vi "Check For Errors.vi"(8 "Error In":errorcluster, 11 "Process In":refnum<class "Process.lvclass">) -> (0 "Error Out":errorcluster, 2 "Error Detected":bool, 3 "Process Out":refnum<class "Process.lvclass">)   [LabVIEW 2021, in "Process.lvclass"]
uses:
  Process.lvclass
  Central Message Handler/Public/Controls/Message.ctl
  Central Message Handler/Central Message Handler.lvclass
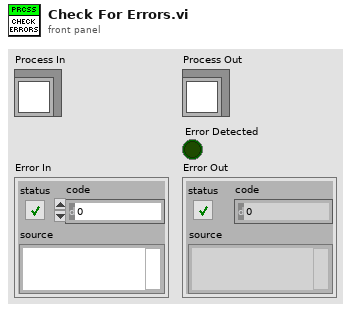
[diagram p1: front panel]
types:
  T1 = typedef "Central Message Handler.lvclass/Message.ctl" = cluster{"Command":string, "Data":variant, "Receiver":string}
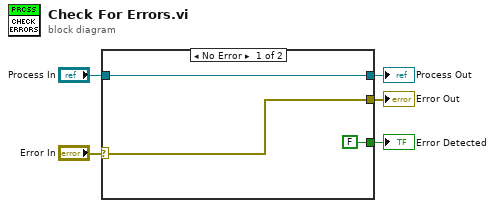
[diagram p0: block diagram]
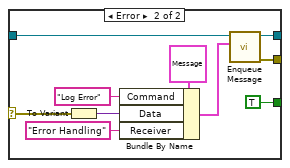
[diagram p2: hidden frame]
diagram:
  n1 = case shown="No Error" "Error In" {
    selector: "Error In" -> [w7 w15]
    tunnel: [w7 w10] -> w4
    tunnel: "Process In" -> [w8 w18]
    tunnel: [w8 w11] -> w2
    tunnel: [FALSE TRUE] -> w1
    frame No Error {
    }
    frame Error {
      n2 = To Variant(anything=w15) -> (Variant=w16:variant)
      n3 = Bundle By Name(cluster=T1 {"Command"="", "Data"=variant, "Receiver"=""} ("element"), "Command"="Log Error", "Data"=w16, "Receiver"="Error Handling") -> (w12:T1)
      n4 = call "Enqueue Message.vi"("Message"=w12, "Process In"=w18) -> ("Error Out"=w10:errorcluster, "Process Out"=w11:refnum<class "Process.lvclass">)  [unwired: 8 in]
    }
  }
  "Process Out" <- w2
  "Error Out" <- w4
  "Error Detected" <- w1
